vi "Bycicle model (bvs).vi"(3 "Wheel angle (deg)":dbl, 4 "Ground speed (km/h)":dbl, 5 "dt (s)":dbl) -> (0 "New Vehicle Orientation Beta":dbl format="%.2f", 1 "New position Y":dbl format="%.2f", 2 "New position X":dbl format="%.2f")   [LabVIEW 2022 SP3]
panel:
  out "output variable":dbl
  out "Eta":dbl
  out "r":dbl
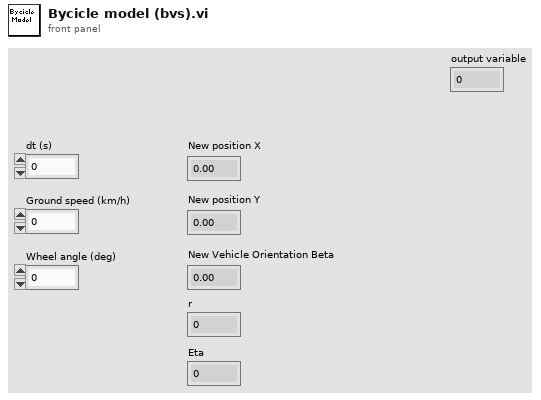
[diagram p1: front panel]
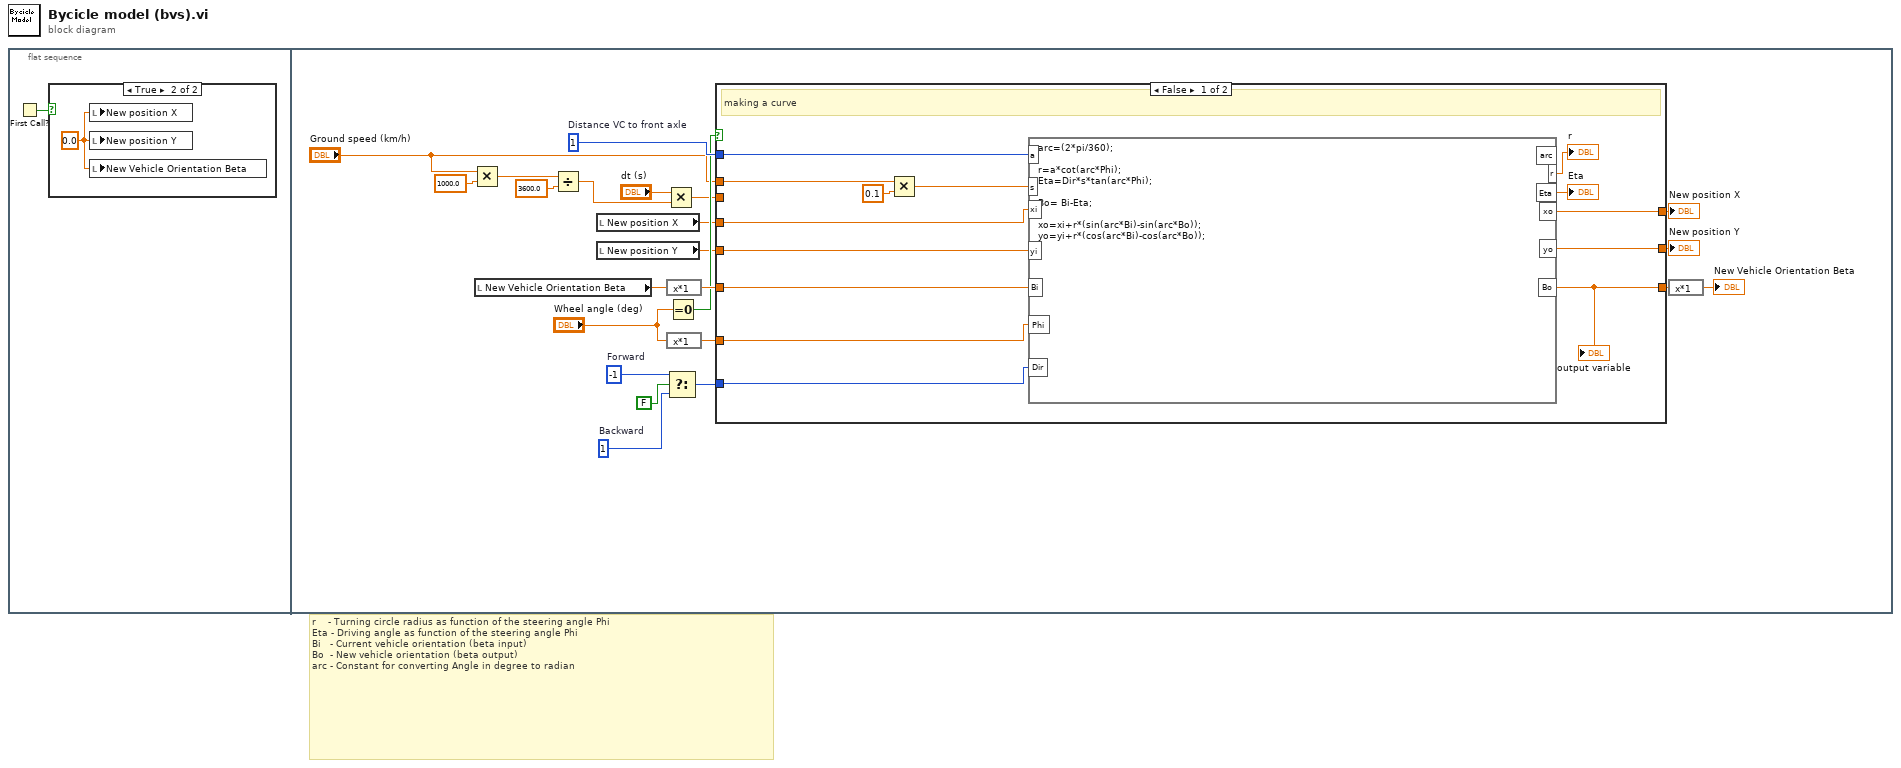
[diagram p0: block diagram]
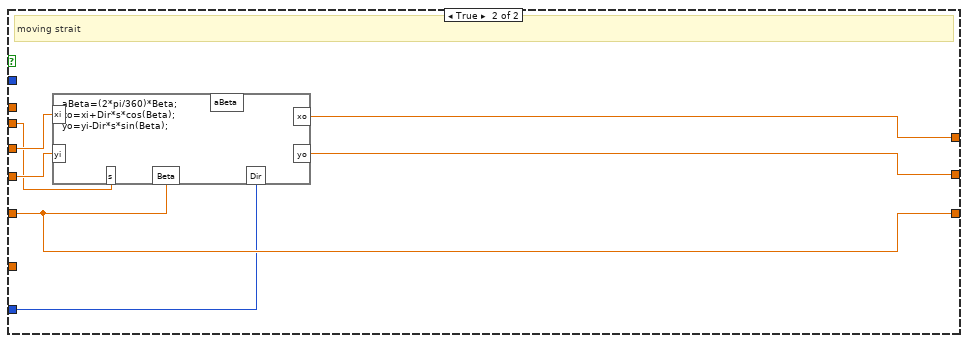
[diagram p3: hidden frame]
diagram:
  # "r    - Turning circle radius as function of the steering angle Phi\nEta - Driving angle as function of the steering angle Phi\nBi   - Current vehicle orientation (beta input)\nBo  - New vehicle orientation (beta output)\narc - Constant for converting Angle in degree to radian"
  n1 = flat-sequence {
    frame #0 {
      n2 = First Call?() -> (First Call?: T/F=w1:bool)
      n3 = case shown="True" w1 {
        frame False {
        }
        frame True {
          w2 = 0.0 ("New position X")
          n4 = local write "New position X"(w2) -> ()
          n5 = local write "New position Y"(w2) -> ()
          n6 = local write "New Vehicle Orientation Beta"(w2) -> ()
        }
      }
    }
    frame #1 {
      w20 = 1  # Distance VC to front axle
      w14 = -1  # Forward
      w15 = 1  # Backward
      n7 = Multiply(x="Ground speed (km/h)", y=1000.0) -> (x*y=w22:dbl)
      n8 = local read "New Vehicle Orientation Beta"() -> (w6:dbl)
      n9 = Divide(x=w22, y=3600.0) -> (x/y=w21:dbl)
      n10 = local read "New position X"() -> (w7:dbl)
      n11 = local read "New position Y"() -> (w5:dbl)
      n12 = Multiply(x="dt (s)", y=w21) -> (x*y=w8:dbl)
      n13 = expression code="x*1"(w6) -> (w18:dbl)
      n14 = expression code="x*1"("Wheel angle (deg)") -> (w17:dbl)
      n15 = Select(t=w14, s=FALSE ("Direction"), f=w15) -> (s? t:f=w16:i32)
      n16 = Equal To 0?(x="Wheel angle (deg)") -> (x = 0?=w12:bool)
      n17 = case shown="False" w12 {
        tunnel: w18 -> [w37 w46]
        tunnel: [w33 w46] -> w19
        tunnel: w7 -> [w39 w45]
        tunnel: w5 -> [w38 w44]
        tunnel: [w31 w43] -> w10
        tunnel: [w32 w42] -> w9
        tunnel: w17 -> [w36 _]
        tunnel: w16 -> [w35 w41]
        tunnel: w20 -> [w34 _]
        tunnel: w8 -> [_ w40]
        tunnel: "Ground speed (km/h)" -> [w28 _]
        frame False {
          # "Bo=(((Bi-Eta)>-90)&&((Bi-Eta)<270)) ? Bi-Eta : ((Bi-Eta)<-90) ? Bi-Eta+360 : Bi-Eta-360;"
          # "making a curve"
          n18 = Multiply(x=w28, y=0.1) -> (x*y=w27:dbl)
          n19 = formula code="arc=(2*pi/360);\n\nr=a*cot(arc*Phi);\nEta=Dir*s*tan(arc*Phi);\n\nBo= Bi-Eta;\n\nxo=xi+r*(sin(arc*Bi)-sin(arc*Bo));\nyo=yi+r*(cos(arc*Bi)-cos(arc*Bo));"("xi"=w39, "yi"=w38, "Bi"=w37, "Phi"=w36, "a"=w34, "Dir"=w35, "s"=w27) -> ("r"=→"r":dbl, "yo"=w32:dbl, "Bo"=w33:dbl, "Eta"=→"Eta":dbl, "xo"=w31:dbl)  [unwired: 1 out]
          "output variable" <- w33
        }
        frame True {
          # "moving strait"
          n20 = formula code="aBeta=(2*pi/360)*Beta;\nxo=xi+Dir*s*cos(Beta);\nyo=yi-Dir*s*sin(Beta);"("xi"=w45, "yi"=w44, "s"=w40, "Beta"=w46, "Dir"=w41) -> ("xo"=w43:dbl, "yo"=w42:dbl)  [unwired: 1 out]
        }
      }
      "New position X" <- w10
      "New position Y" <- w9
      n21 = expression code="x*1"(w19) -> (→"New Vehicle Orientation Beta":dbl)
    }
  }
